vi "Vision - Get all Images for ThumbNail.vi"(6 "ThumbNail Dims":T1, 7 "Printing Report?":bool, 8 "error in (no error)":errorcluster, 9 "Image Distances":dbl[](array[numeric]), 10 "ImagePaths":path[](array[path]), 11 "Image ThumbNails":refnum<vi>) -> (0 "error out":errorcluster, 2 "Rectangle":T2)   [LabVIEW 2024]
uses:
  Controls/ThumbNail Dimensions.ctl
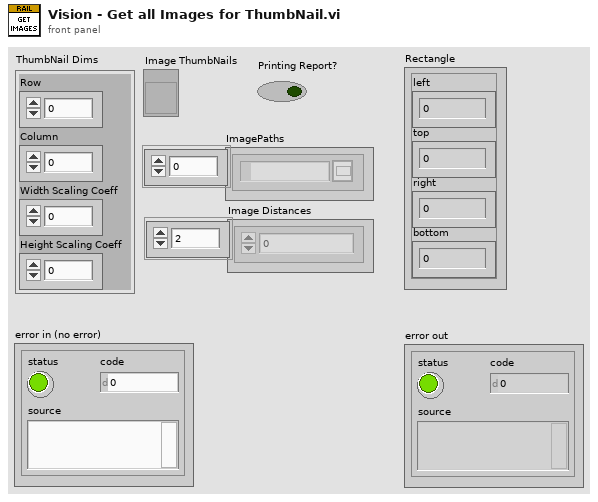
[diagram p1: front panel]
types:
  T1 = typedef "ThumbNail Dimensions.ctl" = cluster{"Row":i32, "Column":i32, "Width Scaling Coeff":dbl, "Height Scaling Coeff":dbl}
  T2 = cluster{"left":i16, "top":i16, "right":i16, "bottom":i16}
  T3 = cluster{"Left Picture":picture, "Distance":string}
  T4 = typedef "imagedata.ctl" = cluster{"image type":i32, "image depth":i32, "image":u8[], "mask":u8[], "colors":u32[], "Rectangle":cluster{"left":i16, "top":i16, "right":i16, "bottom":i16}}
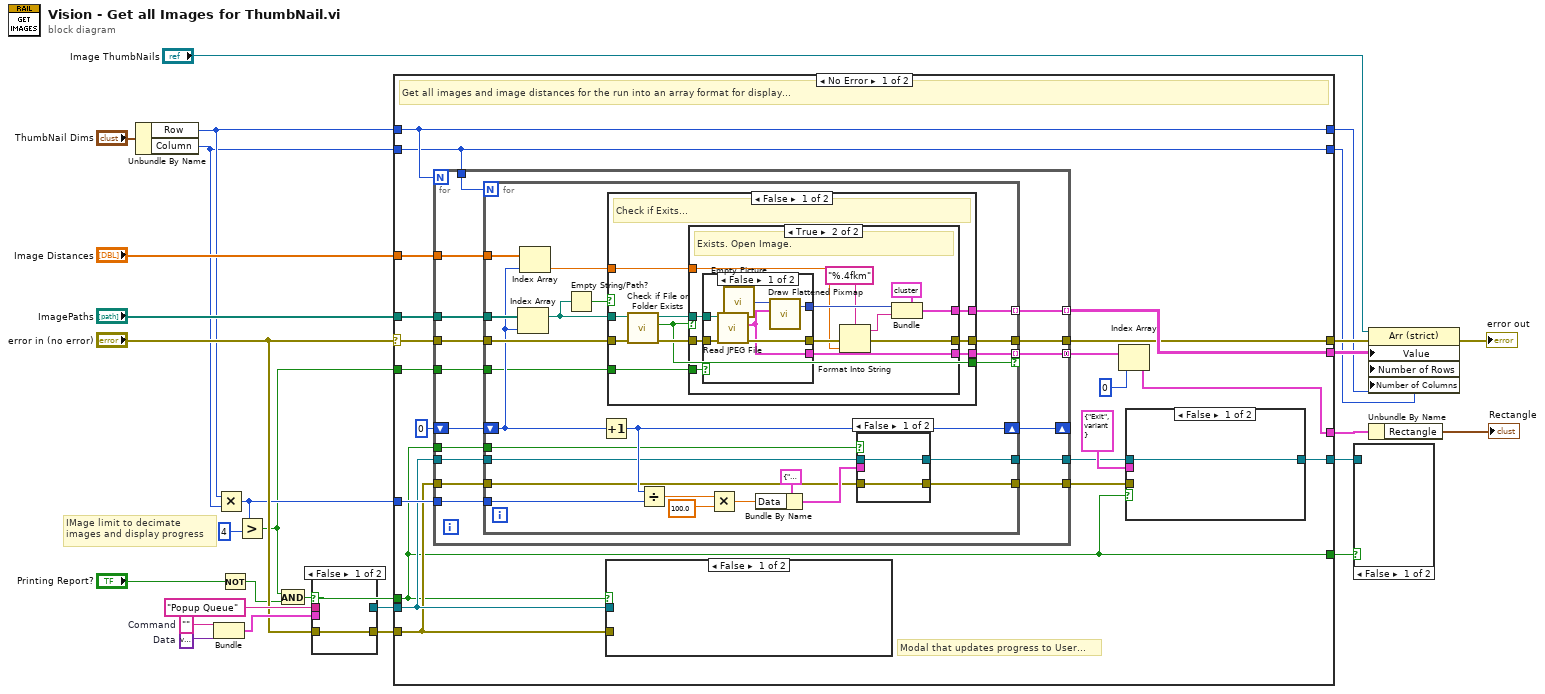
[diagram p0: block diagram]
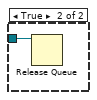
[diagram p2: hidden frame]
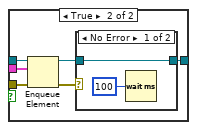
[diagram p3: hidden frame]
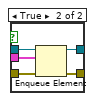
[diagram p5: hidden frame]
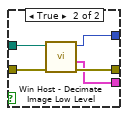
[diagram p7: hidden frame]
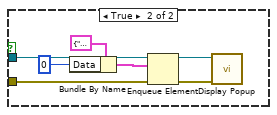
[diagram p9: hidden frame]
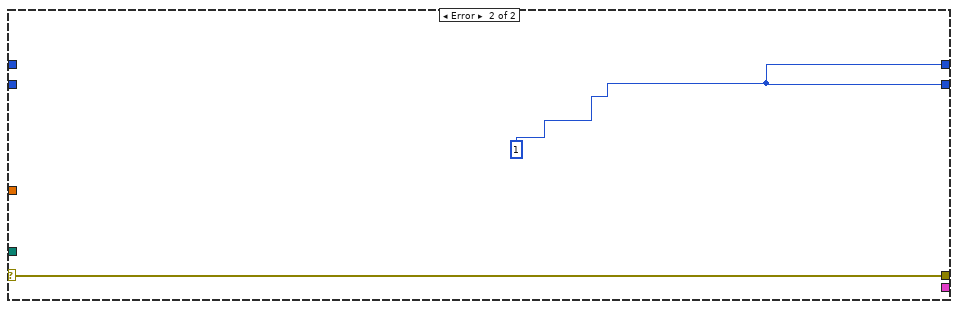
[diagram p10: hidden frame]
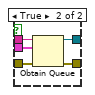
[diagram p11: hidden frame]
diagram:
  w17 = variant  # Data
  w16 = ""  # Command
  # "IMage limit to decimate\nimages and display progress"
  n1 = Unbundle By Name("ThumbNail Dims") -> ("Row"=w2:i32, "Column"=w1:i32)
  n2 = Bundle("Command"=w16, "Data"=w17) -> (w18:cluster{"Command":string, "Data":variant})  [unwired: 1 in]
  n3 = Multiply(x=w2, y=w1) -> (x*y=w10:i32)
  n4 = Not(x="Printing Report?") -> (.not. x?=w4:bool)
  n5 = Greater?(x=w10, y=4) -> (0:w6:bool)
  n6 = And(x=w6, y=w4) -> (x .and. y?=w7:bool)
  n7 = case shown="False" w7 {
    tunnel: w18 -> [_ w34]
    tunnel: "Popup Queue" ("name (unnamed)") -> [_ w33]
    tunnel: "error in (no error)" -> [w29 w32]
    tunnel: [w29 w31] -> w13
    tunnel: [_ w30] -> w11
    frame False {
    }
    frame True {
      n8 = Obtain Queue(name (unnamed)=w33, element data type=w34, error in (no error)=w32) -> (queue out=w30:refnum<queue>, error out=w31:errorcluster)  [unwired: 2 in, 1 out]
    }
  }
  n9 = case shown="No Error" "error in (no error)" {
    selector: "error in (no error)" -> [w51 w155]
    tunnel: [w54 _] -> w28
    tunnel: "ImagePaths" -> [w53 _]
    tunnel: [w47 w155] -> w25
    tunnel: w2 -> [w50 _]
    tunnel: w1 -> [w49 _]
    tunnel: [w50 w154] -> w24
    tunnel: [w49 w154] -> w23
    tunnel: "Image Distances" -> [w48 _]
    tunnel: [w46 _] -> w20
    tunnel: w13 -> [w41 _]
    tunnel: w7 -> [w36 _]
    tunnel: w11 -> [w42 _]
    tunnel: w10 -> [w43 _]
    tunnel: [w37 _] -> w9
    tunnel: [w36 _] -> w8
    tunnel: w6 -> [w35 _]
    frame No Error {
      # "Modal that updates progress to User..."
      # "Get all images and image distances for the run into an array format for display..."
      n10 = for {
        N: w50 -> [_]
        tunnel: [w80] -> w47
        tunnel: [w79] -> w54 mode=indexing
        tunnel: w49 -> [w78]
        shift-right: [w76] -> _
        shift-left: 0 -> [w77]
        tunnel: w53 -> [w75]
        tunnel: w51 -> [w74]
        tunnel: w48 -> [w73]
        tunnel: [w72] -> w45 mode=concatenating
        tunnel: w43 -> [w71]
        tunnel: w42 -> [w70]
        tunnel: w41 -> [w69]
        tunnel: w36 -> [w68]
        tunnel: [w67] -> w39
        tunnel: [w66] -> w38
        tunnel: w35 -> [w65]
        n11 = for {
          N: w78 -> [_]
          tunnel: [w103] -> w80
          tunnel: [w98] -> w79 mode=indexing
          shift-right: [w88] -> w76
          shift-left: w77 -> [w94]
          tunnel: w75 -> [w104]
          tunnel: w74 -> [w100]
          tunnel: w73 -> [w102]
          tunnel: [w99] -> w72 mode=indexing if=w97
          tunnel: w71 -> [w87]
          tunnel: w70 -> [w86]
          tunnel: w69 -> [w85]
          tunnel: w68 -> [w82]
          tunnel: [w84] -> w67
          tunnel: [w83] -> w66
          tunnel: w65 -> [w81]
          n12 = Index Array(array=w104, index=w94) -> (element=w96:path)
          n13 = Index Array(array=w102, index=w94) -> (element=w101:dbl)
          n14 = Empty String/Path?(string/path=w96) -> (empty?=w95:bool)
          n15 = Increment(x=w94) -> (x+1=w88:i32)
          n16 = case shown="False" w95 {
            tunnel: [w121 w146] -> w103
            tunnel: w101 -> [w120 _]
            tunnel: w100 -> [w119 w146]
            tunnel: [w117 _] -> w99
            tunnel: [w116 _] -> w98
            tunnel: [w114 _] -> w97
            tunnel: w96 -> [w113 _]
            tunnel: w81 -> [w112 _]
            frame False {
              # "Check if Exits..."
              n17 = call <vilib>:"Check if File or Folder Exists.vi"("error in (no error)"=w119, "path"=w113) -> ("error out"=w118:errorcluster, "file or folder exists?"=w114:bool, "dup path"=w115:path)  [unwired: 7 in]
              n18 = case shown="True" w114 {
                tunnel: [w122 w127] -> w121
                tunnel: w120 -> [_ w126]
                tunnel: w115 -> [_ w131]
                tunnel: w118 -> [w122 w130]
                tunnel: [_ w129] -> w117
                tunnel: [_ w128] -> w116
                tunnel: w112 -> [_ w123]
                frame False {
                }
                frame True {
                  # "Exists. Open Image."
                  n19 = case shown="False" w123 {
                    tunnel: [w140 w143] -> w133
                    tunnel: [w139 w142] -> w132
                    tunnel: w131 -> [w138 w144]
                    tunnel: w130 -> [w137 w145]
                    tunnel: [w136 w141] -> w129
                    frame False {
                      n20 = call <vilib>:"Read JPEG File.vi"("error in (no error)"=w137, "path to JPEG file"=w138) -> ("error out"=w139:errorcluster, "image data"=w136:T4)  [unwired: 7 in, 1 out]
                      n21 = call "Empty Picture"() -> ("empty picture"=w135:picture)
                      n22 = call <vilib>:"Draw Flattened Pixmap.vi"("image data"=w136, "picture"=w135) -> ("new picture"=w140:picture)  [unwired: 7 in]
                    }
                    frame True {
                      n23 = call "Win Host - Decimate Image Low Level.vi"("error in (no error)"=w145, "Image Path"=w144) -> ("error out"=w142:errorcluster, "ImageData"=w141:T4, "new picture"=w143:picture)  [unwired: 6 in, 1 out]
                    }
                  }
                  n24 = Format Into String(format string="%.4fkm", error in=w132, w126) -> (resulting string=w125:string, error out=w127:errorcluster)  [unwired: 1 in]
                  n25 = Bundle(cluster=T3 {"Left Picture"=bytes[2764830], "Distance"=""} ("Cluster"), "Left Picture"=w133, "Distance"=w125) -> (w128:T3)
                }
              }
            }
            frame True {
            }
          }
          n26 = Divide(x=w88, y=w87) -> (x/y=w92:dbl)
          n27 = Multiply(x=w92, y=100.0) -> (x*y=w91:dbl)
          n28 = Bundle By Name(cluster=cluster{"Command":string, "Data":variant} {"Command"="Update Progress", "Data"=variant} ("output cluster"), "Data"=w91) -> (w93:cluster{"Command":string, "Data":variant})
          n29 = case shown="False" w82 {
            tunnel: w93 -> [_ w111]
            tunnel: w86 -> [w106 w110]
            tunnel: w85 -> [w105 w109]
            tunnel: [w106 w108] -> w84
            tunnel: [w105 w107] -> w83
            frame False {
            }
            frame True {
              n30 = Enqueue Element(queue=w110, element=w111, error in (no error)=w109) -> (queue out=w108:refnum<queue>, error out=w107:errorcluster)  [unwired: 1 in, 1 out]
            }
          }
        }
      }
      n31 = case shown="False" w36 {
        tunnel: w41 -> [_ w148]
        tunnel: w42 -> [_ w147]
        frame False {
        }
        frame True {
          n32 = Bundle By Name(cluster=cluster{"Command":string, "Data":variant} {"Command"="Update Progress", "Data"=variant} ("output cluster"), "Data"=u8 0 ("Progress")) -> (w153:cluster{"Command":string, "Data":variant})
          n33 = Enqueue Element(queue=w147, element=w153, error in (no error)=w148) -> (queue out=w151:refnum<queue>, error out=w152:errorcluster)  [unwired: 1 in, 1 out]
          n34 = call "Display Popup.vi"("error in"=w152, "queue in"=w151) -> ()  [unwired: 8 in, 2 out]
        }
      }
      n35 = Index Array(array=w45, index=0) -> (element=w46:T4)
      n36 = case shown="False" w36 {
        tunnel: cluster{"Command":string, "Data":variant} {"Command"="Exit", "Data"=variant} ("output cluster") -> [_ w61]
        tunnel: w39 -> [w55 w60]
        tunnel: w38 -> [_ w59]
        tunnel: [w55 w57] -> w37
        frame False {
        }
        frame True {
          n37 = Enqueue Element(queue=w60, element=w61, error in (no error)=w59) -> (queue out=w56:refnum<queue>, error out=w58:errorcluster)  [unwired: 1 in, 1 out]
          n38 = case shown="No Error" w58 {
            tunnel: [w62 w64] -> w57
            tunnel: w56 -> [w62 w64]
            frame No Error {
              n39 = Wait (ms)(milliseconds to wait=u32 100) -> ()  [unwired: 1 out]
            }
            frame Error {
            }
          }
        }
      }
    }
    frame Error {
      w154 = 1 ("Rows")
    }
  }
  n40 = case shown="False" w8 {
    tunnel: w9 -> [_ w156]
    frame False {
    }
    frame True {
      n41 = Release Queue(queue=w156) -> ()  [unwired: 2 in, 3 out]
    }
  }
  n42 = property class="Arr (strict)"(reference="Image ThumbNails", error in=w25, "Value"=w28, "Number of Rows"=w24, "Number of Columns"=w23) -> (error out=→"error out":errorcluster)  [unwired: 1 out]
  n43 = Unbundle By Name(w20) -> ("Rectangle"=→"Rectangle":T2)
